vi "create.vi"(8 "error in (no error)":errorcluster, 10 "subpanel":refnum<vi>, 11 "mclb":refnum<vi>) -> (0 "error out":errorcluster, 3 "window":refnum<class "rywindow.lvclass">)   [LabVIEW 2017, in "rywindow.lvclass"]
uses:
  rywindow.lvclass
  data.ctl
  thread.ctl
  <vilib>/Utility/miscctls.llb/LVFontTypeDef.ctl
  rywindow.lvclass/rywindow.ctl
  daemon.vi
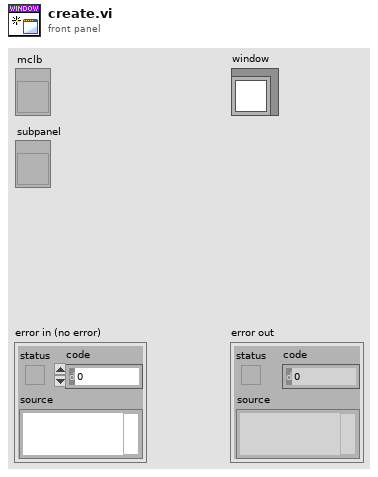
[diagram p1: front panel]
types:
  T1 = typedef "rywindow.lvclass/data.ctl" = cluster{"threads":T2[], "MinSize":cluster{"Width":u32, "Height":u32}, "font":T3, "active":i32}
  T2 = typedef "rywindow.lvclass/thread.ctl" = cluster{"name":string, "vi":refnum<vi>}
  T3 = typedef "LVFontTypeDef.ctl" = cluster{"Font Name":string, "Size":u16, "Bold":bool, "Italic":bool, "Underline":bool, "Strikeout":bool, "Color":u32}
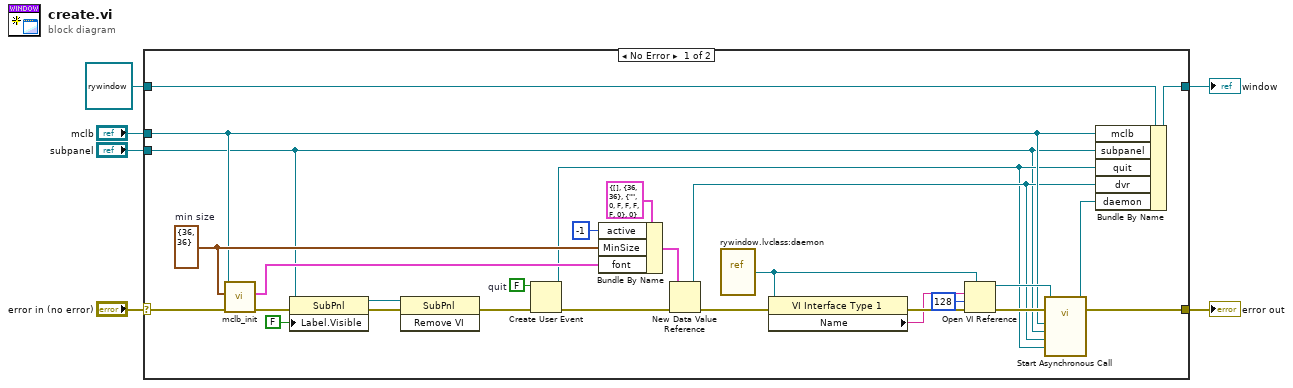
[diagram p0: block diagram]
diagram:
  n1 = case shown="No Error" "error in (no error)" {
    selector: "error in (no error)" -> [w24 w36]
    tunnel: [w17 w36] -> w5
    tunnel: [w32 w35] -> w3
    tunnel: refnum<class "rywindow.lvclass"> refnum ("window in") -> [w34 w35]
    tunnel: "mclb" -> [w15 _]
    tunnel: "subpanel" -> [w9 _]
    frame No Error {
      w25 = FALSE  # quit
      w27 = cluster{"Width":u32, "Height":u32} {"Width"=36, "Height"=36}  # min size
      n2 = call "mclb_init.vi"("error in (no error)"=w24, "min size (36, 36)"=w27, "mclb in"=w15) -> ("error out"=w31:errorcluster, "default font"=w23:T3)  [unwired: 6 in, 1 out]
      n3 = property class="SubPnl"(reference=w9, error in=w31, "Label.Visible"=FALSE) -> (reference out=w8:refnum<vi>, error out=w10:errorcluster)
      n4 = invoke class="SubPnl" method="Remove VI"(reference=w8, error in=w10) -> (error out=w30:errorcluster)  [unwired: 1 in, 2 out]
      n5 = Create User Event(user event datatype=w25, error in=w30) -> (user event=w13:refnum<user-event>, error out=w26:errorcluster)
      n6 = Bundle By Name(cluster=T1 {"threads"=[], "MinSize"={"Width"=36, "Height"=36}, "font"={"Font Name"="", "Size"=0, "Bold"=FALSE, "Italic"=FALSE, "Underline"=FALSE, "Strikeout"=FALSE, "Color"=0}, "active"=0} ("data"), "active"=-1, "MinSize"=w27, "font"=w23) -> (w28:T1)
      n7 = New Data Value Reference(data value=w28, error in=w26) -> (data value reference=w14:refnum<data-value>, error out=w33:errorcluster)
      n8 = vi-ref "rywindow.lvclass:daemon.vi"() -> (w20:refnum<vi>)
      n9 = property class="VI Interface Type 1"(reference=w20, error in=w33) -> (error out=w21:errorcluster, "Name"=w19:string)  [unwired: 1 out]
      n10 = Open VI Reference(type specifier VI Refnum (for type only)=w20, vi path=w19, options=128, error in (no error)=w21) -> (vi reference=w16:refnum<vi>, error out=w22:errorcluster)  [unwired: 2 in]
      n11 = call-by-ref "Start Asynchronous Call"(reference=w16, error in=w22, "quit"=w13, "dvr"=w14, "subpanel"=w9, "mclb"=w15) -> (reference out=w11:refnum<vi>, error out=w17:errorcluster)  [unwired: 8 in]
      n12 = Bundle By Name(cluster=w34, "mclb"=w15, "subpanel"=w9, "quit"=w13, "dvr"=w14, "daemon"=w11) -> (w32:refnum<class "rywindow.lvclass">)
    }
    frame Error {
    }
  }
  "error out" <- w5
  "window" <- w3
